vi "ValueExist.vi"(8 "error in (no error)":errorcluster caption="错误输入（无错误）", 10 "Value":variant, 11 "HashTable 输入":refnum<class "HashTable.lvclass"> caption="DNL_LabVIEW Object in") -> (0 "error out":errorcluster caption="错误输出", 2 "ContainsValue":bool, 3 "HashTable 输出":refnum<class "HashTable.lvclass"> caption="DNL_LabVIEW Object out")   [LabVIEW 2012, in "HashTable.lvclass"]
uses:
  HashTable.lvclass
  HashTable.lvclass/HashTable.ctl
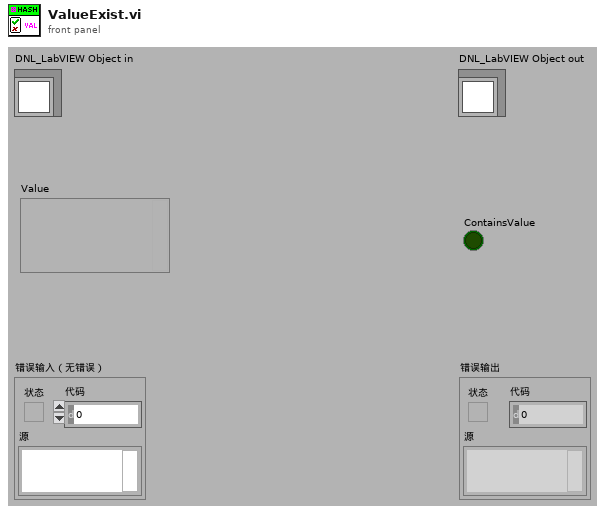
[diagram p1: front panel]
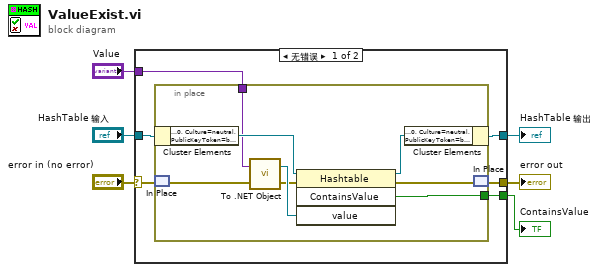
[diagram p0: block diagram]
diagram:
  n1 = case shown="无错误" "error in (no error)" {
    selector: "error in (no error)" -> [w11 w22]
    tunnel: [w10 w22] -> w5
    tunnel: [w7 w21] -> w3
    tunnel: "HashTable 输入" -> [w12 w21]
    tunnel: "Value" -> [w9 _]
    tunnel: [w8 _] -> w1
    frame No Error {
      n2 = in-place {
        in-place-border: w9 -> [w17]
        in-place-border: [w13] -> w8
        n3 = in-place-cluster #1(w12) -> ("HashTable"=w20:refnum<k24>)
        n4 = in-place-match #2(w11) -> (w16:errorcluster)
        n5 = call <vilib>:"To .NET Object.vi"("error in (no error)"=w16, "anything"=w17) -> ("error out"=w15:errorcluster, ".NET object"=w18:refnum<k24>)
        n6 = invoke class="Hashtable" method="ContainsValue"(reference=w20, error in=w15, "value"=w18) -> (reference out=w19:refnum<k24>, error out=w14:errorcluster, "ContainsValue"=w13:bool)  [unwired: 1 in, 1 out]
        n7 = in-place-cluster #1("HashTable"=w19) -> (w7:refnum<class "HashTable.lvclass">)
        n8 = in-place-match #2(w14) -> (w10:errorcluster)
      }
    }
    frame Error {
    }
  }
  "error out" <- w5
  "HashTable 输出" <- w3
  "ContainsValue" <- w1
